vi "MM9.InitDataColl.vi"(0 "i ref in":refnum<vi>, 3 "ms timeout (10000)":i32=10000, 5 "error in (no error)":errorcluster) -> (14 "i ref out":refnum<vi>, 17 "timed out":bool, 19 "error out":errorcluster)   [LabVIEW 2014, in "MM9.lvlib"]
doc: "initializes the data collector."
uses:
  MM9.lvlib
  CSCore/CSSystem/CoreLib/CoreLib.string 2 byte array.vi
  CSCore/CSSystem/CoreLib/CoreLib.lvlib
  CSCore/BaseProcess/BaseProcess.lvlib
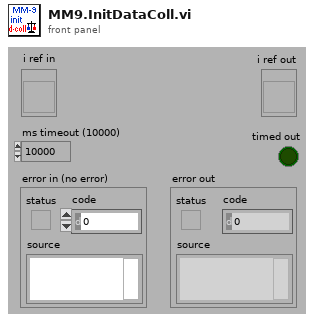
[diagram p1: front panel]
types:
  T1 = typedef "CoreDefs.rawDataType.ctl" = i8[]
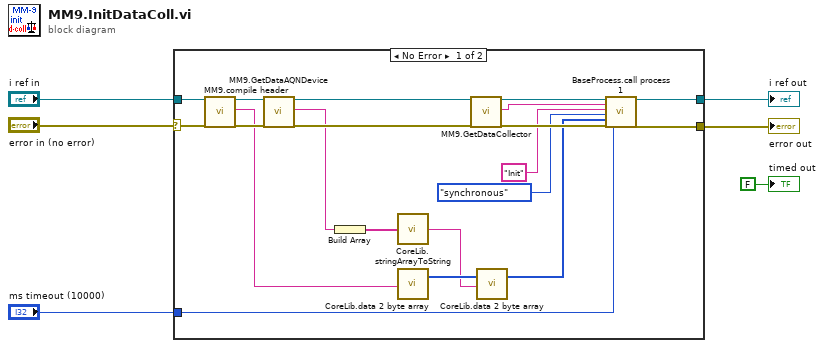
[diagram p0: block diagram]
diagram:
  n1 = case shown="No Error" "error in (no error)" {
    selector: "error in (no error)" -> [w10 w27]
    tunnel: "i ref in" -> [w11 w28]
    tunnel: [w22 w27] -> w4
    tunnel: [w21 w28] -> w3
    tunnel: "ms timeout (10000)" -> [w16 _]
    frame No Error {
      n2 = call "MM9.compile header.vi"("i ref in"=w11, "error in (no error)"=w10) -> ("i ref out"=w9:refnum<vi>, "my header"=w7:string, "error out"=w8:errorcluster)  [unwired: 15 in]
      n3 = call "MM9.GetDataAQNDevice.vi"("i ref in"=w9, "error in (no error)"=w8) -> ("i ref out"=w24:refnum<vi>, "ConfigData.MCA.Name"=w18:string, "error out"=w23:errorcluster)  [unwired: 15 in]
      n4 = Build Array(w18) -> (w17:string[])
      n5 = call "CoreLib.stringArrayToString.vi"("Array"=w17) -> ("String"=w19:string)
      n6 = call-poly "CoreLib.data 2 byte array.vi"("string"=w7) -> ("byteArray out"=w20:T1)  [unwired: 18 in]
      n7 = call "MM9.GetDataCollector.vi"("i ref in"=w24, "error in (no error)"=w23) -> ("i ref out"=w26:refnum<vi>, "data collector"=w15:string, "error out"=w25:errorcluster)  [unwired: 15 in]
      n8 = call-poly "CoreLib.data 2 byte array.vi"("byteArray"=w20, "string"=w19) -> ("byteArray out"=w12:T1)  [unwired: 17 in]
      n9 = call "BaseProcess.call process 1.vi"("i ref in"=w26, "Object"=w15, "Selector"="Init", "CallType"=enum16{"simple", "synchronous", "asynchronous"}."synchronous", "Data"=w12, "error in (no error)"=w25, "timeout (ms)"=w16) -> ("i ref out"=w21:refnum<vi>, "error out"=w22:errorcluster)  [unwired: 10 in, 1 out]
    }
    frame Error {
    }
  }
  "error out" <- w4
  "i ref out" <- w3
  "timed out" <- FALSE ("timed out")
